vi "ParseFormula_RR.vi"(3 "Script":string) -> (1 "URAPI":string)   [LabVIEW 2012]
panel:
  out "Cleaned up script":string
  out "Array":string[](array[string])
  # "a +(b -(c * d))"
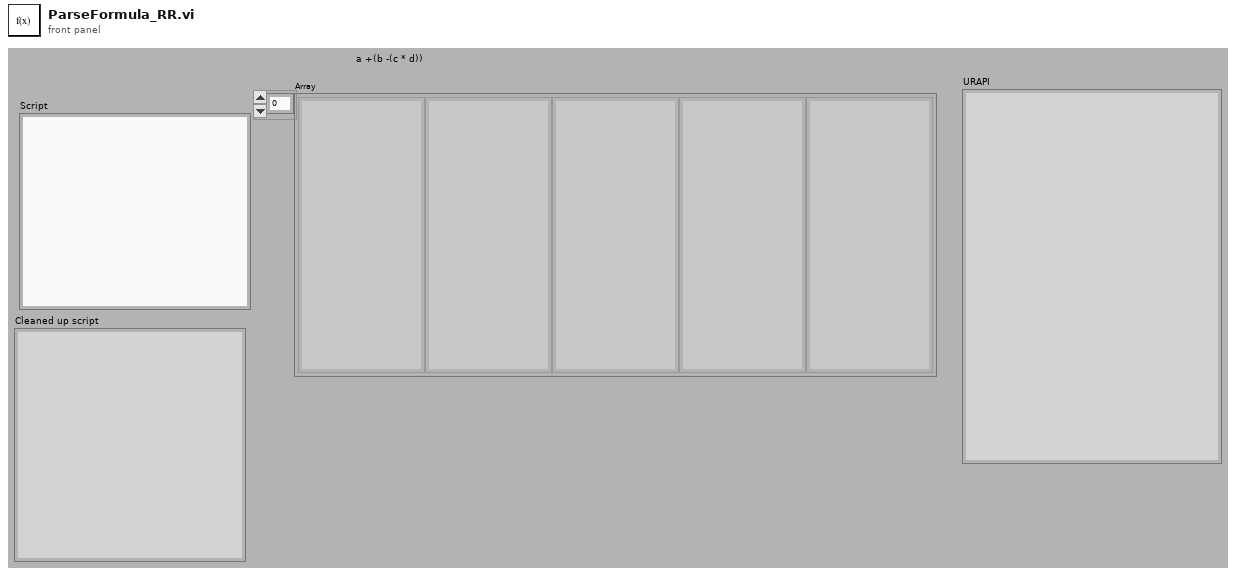
[diagram p1: front panel]
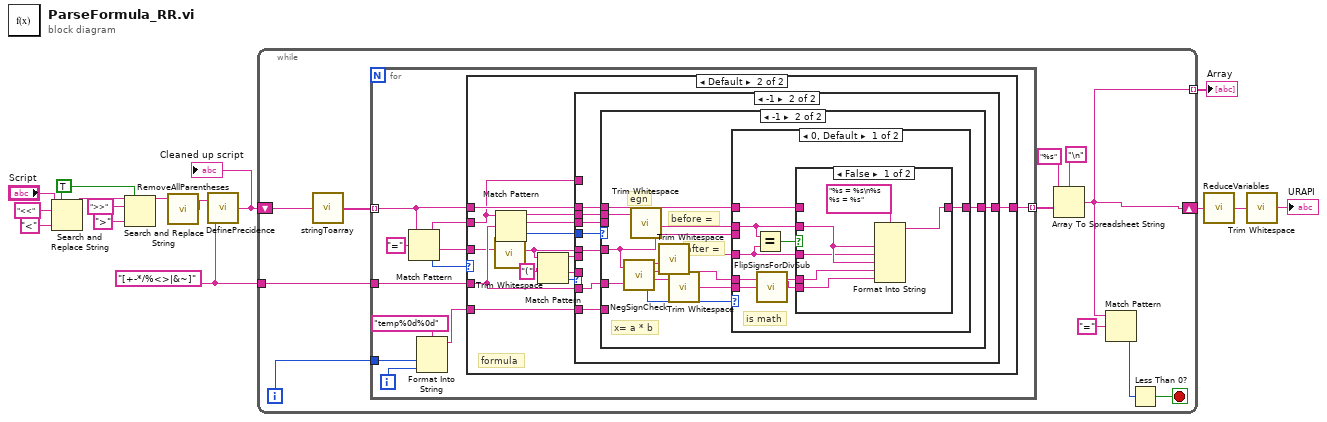
[diagram p0: block diagram]
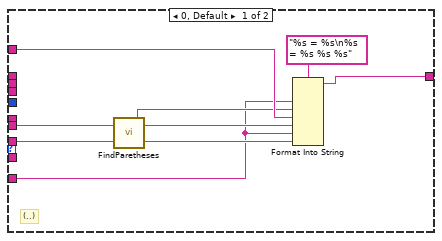
[diagram p3: hidden frame]
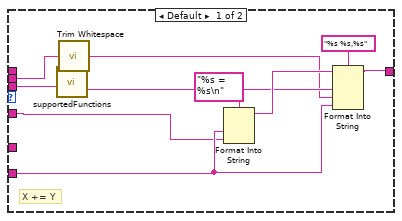
[diagram p4: hidden frame]
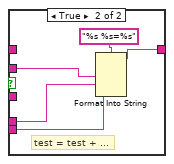
[diagram p5: hidden frame]
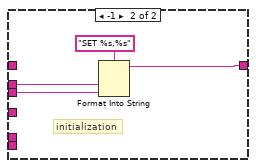
[diagram p6: hidden frame]
diagram:
  w2 = TRUE ("replace all? (F)")
  w12 = "[+-*/%<>|&~]" ("regular expression")
  n1 = Search and Replace String(replace all?=w2, input string="Script", search string="<<", replace string="<" ("replace string (\"\")")) -> (result string=w4:string)  [unwired: 4 in, 3 out]
  n2 = Search and Replace String(replace all?=w2, input string=w4, search string=">>", replace string=">" ("replace string (\"\")")) -> (result string=w3:string)  [unwired: 4 in, 3 out]
  n3 = call <userlib>:"RemoveAllParentheses.vi"("Script in"=w3) -> ("Script out"=w10:string)
  n4 = call <userlib>:"DefinePrecidence.vi"("regular expression"=w12, "Script in"=w10) -> ("Script out"=w11:string)
  "Cleaned up script" <- w11
  n5 = while {
    shift-right: [w20] -> w13
    shift-left: w11 -> [w17]
    tunnel: [w20] -> w15 mode=indexing
    tunnel: w12 -> [w19]
    i -> [w16]
    stop <- w21 stop-if-true
    n6 = call <userlib>:"stringToarray.vi"("String"=w17) -> ("Array"=w18:string[])
    n7 = for {
      tunnel: w18 -> [w33] mode=indexing
      tunnel: [w34] -> w26 mode=indexing
      tunnel: w19 -> [w31]
      tunnel: w16 -> [w28]
      i -> [w27]
      n8 = Match Pattern(string=w33, regular expression="=") -> (before substring=w36:string, after substring=w35:string, offset past match=w32:i32)  [unwired: 1 in, 1 out]
      n9 = Format Into String(format string="temp%0d%0d" ("Script"), w28, w27) -> (resulting string=w29:string)  [unwired: 2 in, 1 out]
      n10 = case shown="Default" w32 {
        tunnel: w36 -> [_ w41]
        tunnel: w35 -> [_ w45]
        tunnel: [w38 w52] -> w34
        tunnel: w33 -> [w38 w51]
        tunnel: w31 -> [_ w50]
        tunnel: w29 -> [_ w46]
        frame -1 {
          # "Not a formula"
        }
        frame Default {
          # "formula"
          n11 = call <vilib>:"Trim Whitespace.vi"("string"=w45) -> ("trimmed string"=w44:string)  [unwired: 1 in]
          n12 = Match Pattern(string=w41, regular expression=w50) -> (before substring=w48:string, match substring=w47:string, offset past match=w49:i32)  [unwired: 1 in, 1 out]
          n13 = Match Pattern(string=w44, regular expression="(") -> (before substring=w40:string, after substring=w39:string, offset past match=w43:i32)  [unwired: 1 in, 1 out]
          n14 = case shown="-1" w43 {
            tunnel: [w53 w68] -> w52
            tunnel: w51 -> [_ w67]
            tunnel: w50 -> [_ w66]
            tunnel: w49 -> [_ w65]
            tunnel: w48 -> [_ w64]
            tunnel: w47 -> [_ w63]
            tunnel: w46 -> [w54 w62]
            tunnel: w44 -> [_ w61]
            tunnel: w41 -> [w59 _]
            tunnel: w40 -> [w58 _]
            tunnel: w39 -> [w57 _]
            frame 0, Default {
              # "(..)"
              n15 = call <userlib>:"FindParetheses.vi"("String in"=w57) -> ("rest"=w56:string, "parentetical"=w55:string)
              n16 = Format Into String(format string="%s = %s\n%s = %s %s %s", w54, w55, w59, w58, w54, w56) -> (resulting string=w53:string)  [unwired: 2 in, 1 out]
            }
            frame -1 {
              n17 = case shown="-1" w65 {
                tunnel: w61 -> [w69 w84]
                tunnel: [w75 w89] -> w68
                tunnel: w67 -> [_ w88]
                tunnel: w66 -> [_ w82]
                tunnel: w64 -> [w76 w86]
                tunnel: w63 -> [w78 _]
                tunnel: w62 -> [w73 _]
                frame Default {
                  # "X += Y"
                  n18 = call <userlib>:"supportedFunctions.vi"("String"=w78) -> ("regular expression"=w72:string)  [unwired: 1 out]
                  n19 = call <vilib>:"Trim Whitespace.vi"("string"=w76) -> ("trimmed string"=w71:string)  [unwired: 1 in]
                  n20 = Format Into String(format string="%s = %s\n", w73, w69) -> (resulting string=w74:string)  [unwired: 2 in, 1 out]
                  n21 = Format Into String(format string="%s %s,%s", initial string=w74, w72, w71, w73) -> (resulting string=w75:string)  [unwired: 1 in, 1 out]
                }
                frame -1 {
                  # "after ="
                  # "before ="
                  # "egn"
                  # "x= a * b"
                  n22 = call <userlib>:"NegSignCheck.vi"("regular expression"=w82, "trimmed string"=w84) -> ("offset past match"=w83:i32, "cc"=w79:string, "bb"=w80:string, "aa"=w81:string)
                  n23 = call <vilib>:"Trim Whitespace.vi"("string"=w86) -> ("trimmed string"=w90:string)  [unwired: 1 in]
                  n24 = call <vilib>:"Trim Whitespace.vi"("string"=w81) -> ("trimmed string"=w87:string)  [unwired: 1 in]
                  n25 = call <vilib>:"Trim Whitespace.vi"("string"=w79) -> ("trimmed string"=w85:string)  [unwired: 1 in]
                  n26 = case shown="0, Default" w83 {
                    tunnel: w90 -> [w95 w112]
                    tunnel: w84 -> [_ w111]
                    tunnel: [w97 w110] -> w89
                    tunnel: w88 -> [w96 _]
                    tunnel: w87 -> [w94 _]
                    tunnel: w80 -> [w93 _]
                    tunnel: w85 -> [w92 _]
                    frame 0, Default {
                      # "is math"
                      n27 = Equal?(x=w95, y=w94) -> (x = y?=w98:bool)
                      n28 = call <userlib>:"FlipSignsForDivSub.vi"("RHS"=w92, "operation"=w93) -> ("RHS fixed"=w91:string)  [unwired: 1 in]
                      n29 = case shown="False" w98 {
                        tunnel: [w99 w108] -> w97
                        tunnel: w96 -> [_ _]
                        tunnel: w95 -> [w103 w107]
                        tunnel: w93 -> [w102 w105]
                        tunnel: w91 -> [w101 w106]
                        tunnel: w94 -> [w100 _]
                        frame False {
                          n30 = Format Into String(format string="%s = %s\n%s %s = %s", w103, w100, w103, w102, w101) -> (resulting string=w99:string)  [unwired: 2 in, 1 out]
                        }
                        frame True {
                          # "test = test + ..."
                          n31 = Format Into String(format string="%s %s=%s", w107, w105, w106) -> (resulting string=w108:string)  [unwired: 2 in, 1 out]
                        }
                      }
                    }
                    frame -1 {
                      # "initialization"
                      n32 = Format Into String(format string="SET %s,%s", w112, w111) -> (resulting string=w110:string)  [unwired: 2 in, 1 out]
                    }
                  }
                }
              }
            }
          }
        }
      }
    }
    n33 = Array To Spreadsheet String(delimiter (Tab)="\n", array=w26, 3:"%s" ("delimiter (Tab)")) -> (spreadsheet string=w20:string)
    n34 = Match Pattern(string=w20, regular expression="=") -> (offset past match=w22:i32)  [unwired: 1 in, 3 out]
    n35 = Less Than 0?(x=w22) -> (x < 0?=w21:bool)
  }
  "Array" <- w15
  n36 = call <userlib>:"ReduceVariables.vi"("Script in"=w13) -> ("Script out"=w14:string)
  n37 = call <vilib>:"Trim Whitespace.vi"("string"=w14) -> ("trimmed string"=→"URAPI":string)  [unwired: 1 in]
